vi "Get Point of reflection.vi"(10 "Start point":u64, 11 "Array in":u32[](array[numeric])) -> (3 "Numeric":u64)   [LabVIEW 2020, in "Group.lvclass"]
uses:
  Group.lvclass
  Group.lvclass/Group.ctl
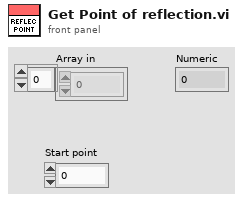
[diagram p1: front panel]
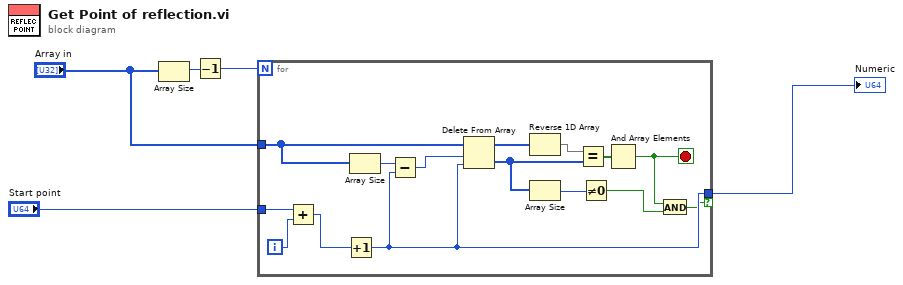
[diagram p0: block diagram]
diagram:
  n1 = Array Size(array="Array in") -> (size(s)=w3:i32)
  n2 = Decrement(x=w3) -> (x-1=w4:i32)
  n3 = for {
    N: w4 -> [_]
    tunnel: "Array in" -> [w17]
    tunnel: [w14] -> w5 if=w7
    tunnel: "Start point" -> [w12]
    i -> [w10]
    stop <- w13 stop-if-true
    n4 = Add(x=w12, y=w10) -> (x+y=w11:u64)
    n5 = Increment(x=w11) -> (x+1=w14:u64)
    n6 = Array Size(array=w17) -> (size(s)=w16:i32)
    n7 = Subtract(x=w16, y=w14) -> (x-y=w15:u64)
    n8 = Delete From Array(array=w17, length=w15, index=w14) -> (deleted portion=w9:u32[], array with subset deleted=w20:u32[])
    n9 = Reverse 1D Array(array=w20) -> (reversed array=w19:u32[])
    n10 = Array Size(array=w9) -> (size(s)=w8:i32)
    n11 = Equal?(x=w19, y=w9) -> (x = y?=w18:bool[])
    n12 = Not Equal To 0?(x=w8) -> (x != 0?=w6:bool)
    n13 = And Array Elements(Boolean array=w18) -> (logical AND=w13:bool)
    n14 = And(x=w13, y=w6) -> (x .and. y?=w7:bool)
  }
  "Numeric" <- w5
